vi "Convert Oersted to Tesla.vi"(8 "error in (no error)":errorcluster, 10 "Field (Oe)":dbl, 11 "instrument.PPMS in":refnum<class "instrument.PPMS.lvclass">) -> (0 "error out":errorcluster, 2 "Field (T)":dbl, 3 "instrument.PPMS out":refnum<class "instrument.PPMS.lvclass">)   [LabVIEW 2019, in "instrument.PPMS.lvclass"]
uses:
  instrument.PPMS.lvclass
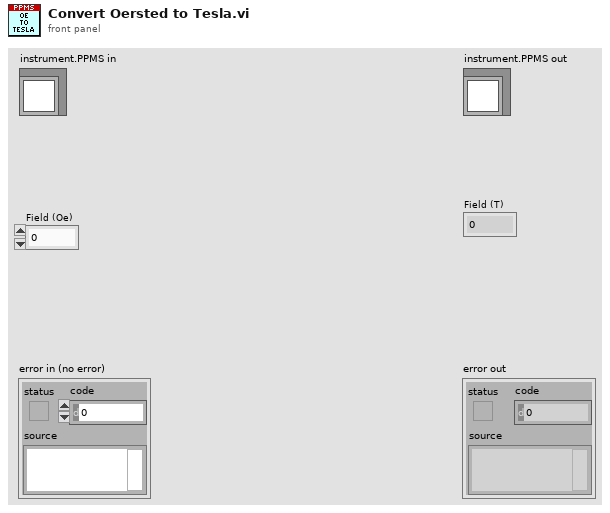
[diagram p1: front panel]
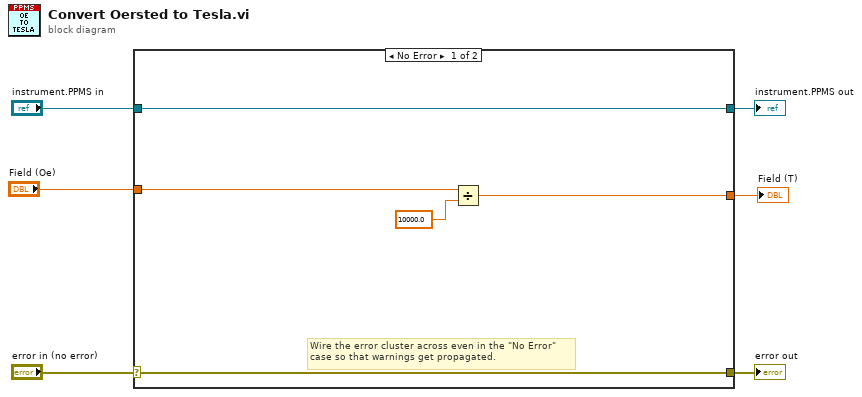
[diagram p0: block diagram]
diagram:
  n1 = case shown="No Error" "error in (no error)" {
    selector: "error in (no error)" -> [w10 w13]
    tunnel: [w10 w13] -> w5
    tunnel: [w11 w12] -> w3
    tunnel: "instrument.PPMS in" -> [w11 w12]
    tunnel: "Field (Oe)" -> [w8 _]
    tunnel: [w7 _] -> w1
    frame No Error {
      # "Wire the error cluster across even in the \"No Error\"\ncase so that warnings get propagated."
      n2 = Divide(x=w8, y=10000.0) -> (x/y=w7:dbl)
    }
    frame Error {
    }
  }
  "error out" <- w5
  "instrument.PPMS out" <- w3
  "Field (T)" <- w1
